vi "Add LargeImages to ListView.vi"(8 "error in (no error)":errorcluster caption="错误输入（无错误）", 10 "LargeImage":path[](array[path]), 11 "ListViewClass 输入":refnum<class "ListViewClass.lvclass"> caption="DNL_LabVIEW Object in") -> (0 "error out":errorcluster caption="错误输出", 3 "ListViewClass 输出":refnum<class "ListViewClass.lvclass"> caption="DNL_LabVIEW Object out")   [LabVIEW 2012, in "ListViewClass.lvclass"]
uses:
  ListViewClass.lvclass
  ListViewClass.lvclass/ListViewClass.ctl
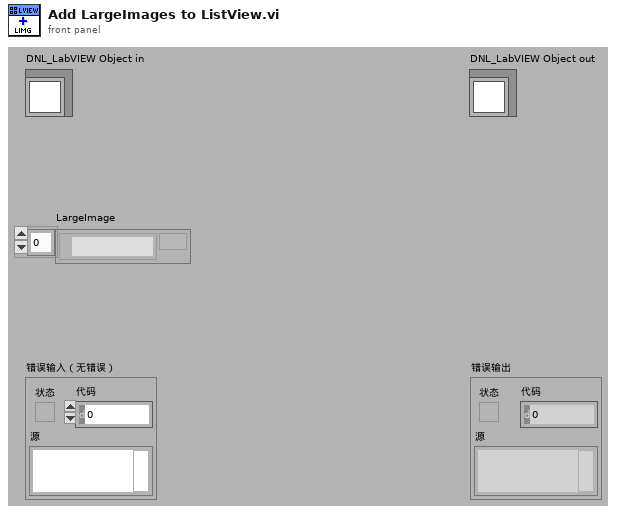
[diagram p1: front panel]
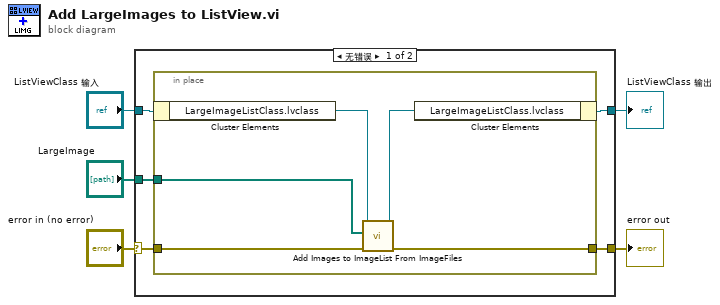
[diagram p0: block diagram]
diagram:
  n1 = case shown="无错误" "error in (no error)" {
    selector: "error in (no error)" -> [w7 w17]
    tunnel: [w6 w17] -> w4
    tunnel: [w9 w16] -> w2
    tunnel: "ListViewClass 输入" -> [w10 w16]
    tunnel: "LargeImage" -> [w8 _]
    frame No Error {
      n2 = in-place {
        in-place-border: w8 -> [w13]
        in-place-border: w7 -> [w12]
        in-place-border: [w11] -> w6
        n3 = in-place-cluster #1(w10) -> ("LargeImageListClass.lvclass"=w15:refnum<class "ImageListClass.lvclass">)
        n4 = call "Add Images to ImageList From ImageFiles.vi"("error in (no error)"=w12, "ImageFile Path"=w13, "ImageListClass 输入"=w15) -> ("error out"=w11:errorcluster, "ImageListClass 输出"=w14:refnum<class "ImageListClass.lvclass">)  [unwired: 7 in]
        n5 = in-place-cluster #1("LargeImageListClass.lvclass"=w14) -> (w9:refnum<class "ListViewClass.lvclass">)
      }
    }
    frame Error {
    }
  }
  "error out" <- w4
  "ListViewClass 输出" <- w2
